vi "Hardware - Counter Time.vi"(7 "Counter Time Function (Read Timer)":T1=enum."Read Timer", 8 "error in (no error)":errorcluster, 11 "Counter Task In":refnum<k21>) -> (0 "error out":errorcluster, 3 "Timer Value (ms)":dbl caption="Time Value (ms)" format="%#.6g")   [LabVIEW 2009, in "Core SubVIs.lvlib"]
uses:
  Core SubVIs.lvlib
  Controls/TYPE - Count Time Method.ctl
  <vilib>/DAQmx/read.llb/DAQmx Read (Counter U32 1Chan 1Samp).vi
  C:/Program Files/National Instruments/LabVIEW 2009/resource/objmgr/daqmx.rc
panel:
  out "HIGH WORD":u32
  in  "Timebase Rate (10 MHz Default)":dbl=10000000.0 format="%#_6p"
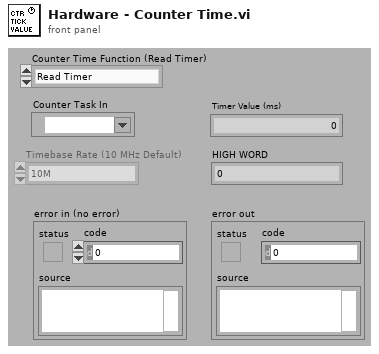
[diagram p1: front panel]
types:
  T1 = typedef "Core SubVIs.lvlib/TYPE - Count Time Method.ctl" = enum16{"Start Timer Task", "Read Timer", "Reset Timer", "Clear Timer Task"}
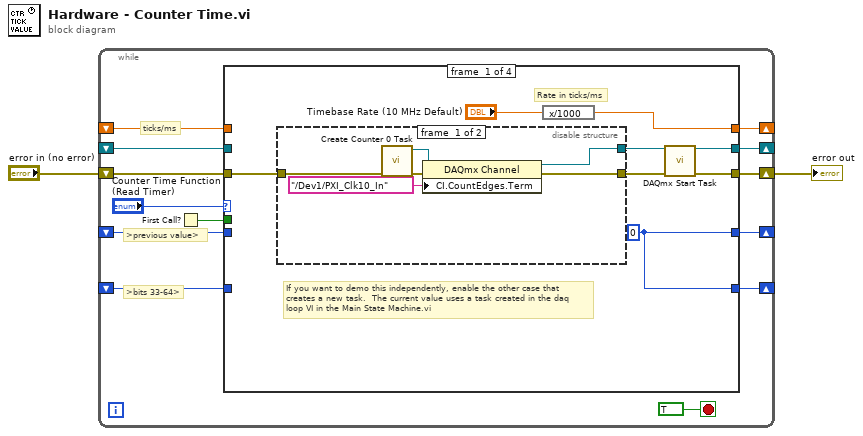
[diagram p0: block diagram]
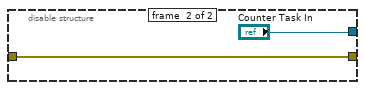
[diagram p2: hidden frame]
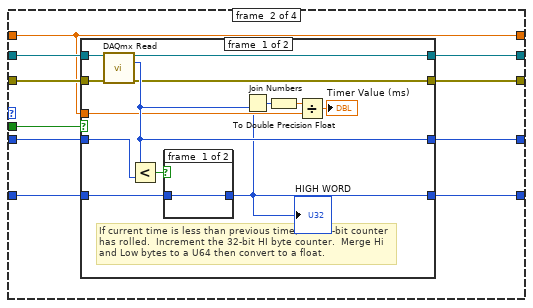
[diagram p3: hidden frame]
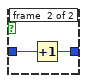
[diagram p4: hidden frame]
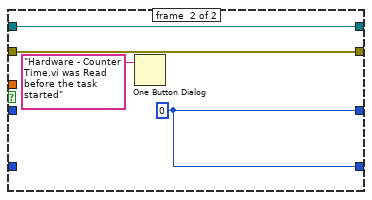
[diagram p5: hidden frame]
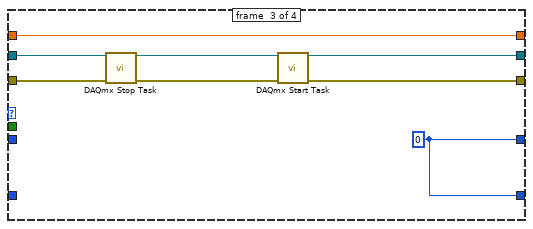
[diagram p6: hidden frame]
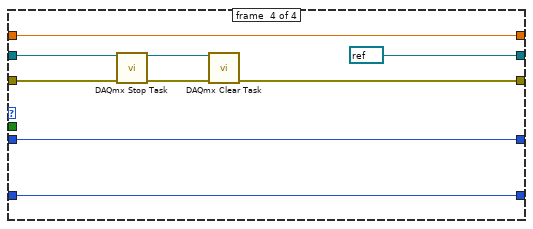
[diagram p7: hidden frame]
diagram:
  n1 = while {
    shift-right: [w12] -> _
    shift-left: _ -> [w15]
    shift-right: [w11] -> w1
    shift-left: "error in (no error)" -> [w14]
    shift-right: [w9] -> _
    shift-left: _ -> [w8]
    shift-right: [w5] -> _
    shift-left: _ -> [w6]
    shift-right: [w3] -> _
    shift-left: _ -> [w4]
    stop <- TRUE stop-if-true
    # ">bits 33-64>"
    # ">previous value>"
    # "ticks/ms"
    n2 = First Call?() -> (First Call?: T/F=w7:bool)
    n3 = case shown="\"Read Timer\"" "Counter Time Function (Read Timer)" {
      tunnel: w15 -> [_ w41 w69 w76]
      tunnel: w14 -> [w20 w40 w68 w75]
      tunnel: [w17 w39 w65 refnum<k21> refnum ("task out")] -> w12
      tunnel: [w18 w38 w64 w74] -> w11
      tunnel: [w22 w32 w63 w72] -> w9
      tunnel: w8 -> [_ w32 w63 w72]
      tunnel: w7 -> [_ w37 _ _]
      tunnel: w6 -> [_ w36 _ w71]
      tunnel: [w21 w35 w62 w71] -> w5
      tunnel: w4 -> [_ w34 _ w70]
      tunnel: [w21 w33 w62 w70] -> w3
      frame #0 {
        w21 = u32 0 ("data")
        # "If you want to demo this independently, enable the other case that\ncreates a new task.  The current value uses a task created in the daq\nloop VI in the Main State Machine.vi"
        # "Rate in ticks/ms"
        n4 = disable-structure shown="Enabled" {
          disable-tunnel: [w24 "Counter Task In"] -> w16
          disable-tunnel: [w25 w30] -> w19
          disable-tunnel: w20 -> [w26 w30]
          frame #0 {
            n5 = call "Create Counter 0 Task.vi"("error in"=w26) -> ("error out"=w27:errorcluster, "task out"=w28:refnum<k21>)  [unwired: 9 in]
            n6 = property class="DAQmx Channel"(reference=w28, error in=w27, "CI.CountEdges.Term"=tag "/Dev1/PXI_Clk10_In") -> (reference out=w24:refnum<k21>, error out=w25:errorcluster)
          }
          frame #1 {
          }
        }
        n7 = expression code="x/1000"("Timebase Rate (10 MHz Default)") -> (w22:dbl)
        n8 = call <vilib>:"DAQmx Start Task.vi"("task/channels in"=w16, "error in"=w19) -> ("task out"=w17:refnum<k21>, "error out"=w18:errorcluster)  [unwired: 12 out]
      }
      frame #1 {
        n9 = case shown="False" w37 {
          tunnel: w41 -> [w52 w61]
          tunnel: w40 -> [w51 w60]
          tunnel: [w50 w61] -> w39
          tunnel: [w49 w60] -> w38
          tunnel: w36 -> [w47 _]
          tunnel: [w54 w58] -> w35
          tunnel: w34 -> [w46 _]
          tunnel: [w42 w58] -> w33
          tunnel: w32 -> [w53 _]
          frame #0 {
            # "If current time is less than previous time, the 32-bit counter has rolled.  Increment the 32-bit HI byte counter.  Merge Hi and Low bytes to a U64 then convert to a float."
            n10 = call-poly <vilib>:"DAQmx Read.vi"("task/channels in"=w52, "error in"=w51) -> ("task out"=w50:refnum<k21>, "data"=w54:u32, "error out"=w49:errorcluster)  [unwired: 1 in, 10 out]
            n11 = Less?(x=w54, y=w47) -> (x < y?=w48:bool)
            n12 = case shown="True" w48 {
              tunnel: w46 -> [w55 w57]
              tunnel: [w55 w56] -> w42
              frame #0 {
              }
              frame #1 {
                n13 = Increment(x=w57) -> (x+1=w56:u32)
              }
            }
            "HIGH WORD" <- w42
            n14 = Join Numbers(hi=w42, lo=w54) -> ((hi.lo)=w45:u64)
            n15 = To Double Precision Float(number=w45) -> (double precision float=w43:dbl)
            n16 = Divide(x=w43, y=w53) -> (x/y=→"Timer Value (ms)":dbl)
          }
          frame #1 {
            w58 = u32 0 ("data")
            n17 = One Button Dialog(message="Hardware - Counter Time.vi was Read before the task started") -> ()  [unwired: 2 out]
          }
        }
      }
      frame #2 {
        w62 = u32 0 ("data")
        n18 = call <vilib>:"DAQmx Stop Task.vi"("task/channels in"=w69, "error in"=w68) -> ("task out"=w67:refnum<k21>, "error out"=w66:errorcluster)  [unwired: 12 out]
        n19 = call <vilib>:"DAQmx Start Task.vi"("task/channels in"=w67, "error in"=w66) -> ("task out"=w65:refnum<k21>, "error out"=w64:errorcluster)  [unwired: 12 out]
      }
      frame #3 {
        n20 = call <vilib>:"DAQmx Stop Task.vi"("task/channels in"=w76, "error in"=w75) -> ("task out"=w77:refnum<k21>, "error out"=w78:errorcluster)  [unwired: 12 out]
        n21 = call <vilib>:"DAQmx Clear Task.vi"("task in"=w77, "error in"=w78) -> ("error out"=w74:errorcluster)  [unwired: 13 out]
      }
    }
  }
  "error out" <- w1
